vi "Allan Variance for range new.vi"(8 "error in (no error)":errorcluster, 10 "n range":i32, 11 "Data in":dbl[](array[numeric])) -> (0 "error out":errorcluster, 2 "Allan Variances":dbl[][](array[numeric]), 3 "Allan Variances graph":cluster{dbl[], dbl[]}(graph))   [LabVIEW 2021]
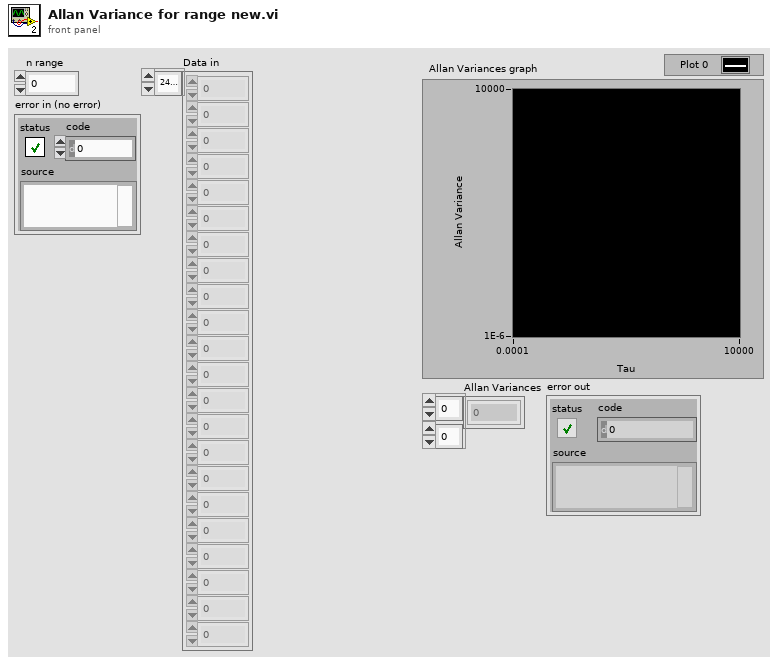
[diagram p1: front panel]
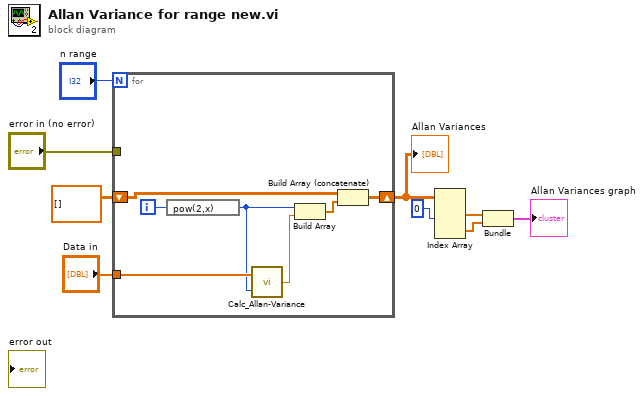
[diagram p0: block diagram]
diagram:
  n1 = for {
    N: "n range" -> [_]
    shift-right: [w16] -> w7
    shift-left: dbl[][] [] -> [w15]
    tunnel: "error in (no error)" -> [_]
    tunnel: "Data in" -> [w12]
    i -> [w13]
    n2 = expression code="pow(2,x)"(w13) -> (w11:i32)
    n3 = call "Calc_Allan-Variance.VI"("tau"=w11, "Input Array"=w12) -> ("Allan-variance (tau)"=w10:dbl)
    n4 = Build Array(w11, w10) -> (w14:dbl[])
    n5 = Build Array (concatenate)(w15, w14) -> (w16:dbl[][])
  }
  "Allan Variances" <- w7
  n6 = Index Array(array=w7, index (col) #1=0 ("disabled index (col)")) -> (element #1=w5:dbl[], element #2=w4:dbl[])  [unwired: 3 in]
  n7 = Bundle(w5, w4) -> (→"Allan Variances graph":cluster{dbl[], dbl[]})  [unwired: 1 in]
